vi "Circle Detection Programmattically.vi"(6 "error in":errorcluster, 8 "File Path":path=path "\\\\WS007462\\Share_Station_20/Dinesh/Electrolux/Level 10_11min_4_0001.JPG", 9 "Color Plane (Color Plane Extraction 1)":i32(ring) items=["Red", "Green", "Blue", "Hue", "Saturation", "Luminance", "Value", "Intensity"]) -> (0 "error out":errorcluster, 1 "Number of Circles detected":i32, 2 "Image Out":T1, 3 "Circles (Shape Detection 1)":T2(array[cluster]) {"Position"."Y" format="%.2f"; "Position"."X" format="%.2f"})   [LabVIEW 2020]
uses:
  <vilib>/vision/NI_Vision_Development_Module.lvlib
  <vilib>/vision/Image Controls.llb/IMAQ Image.ctl
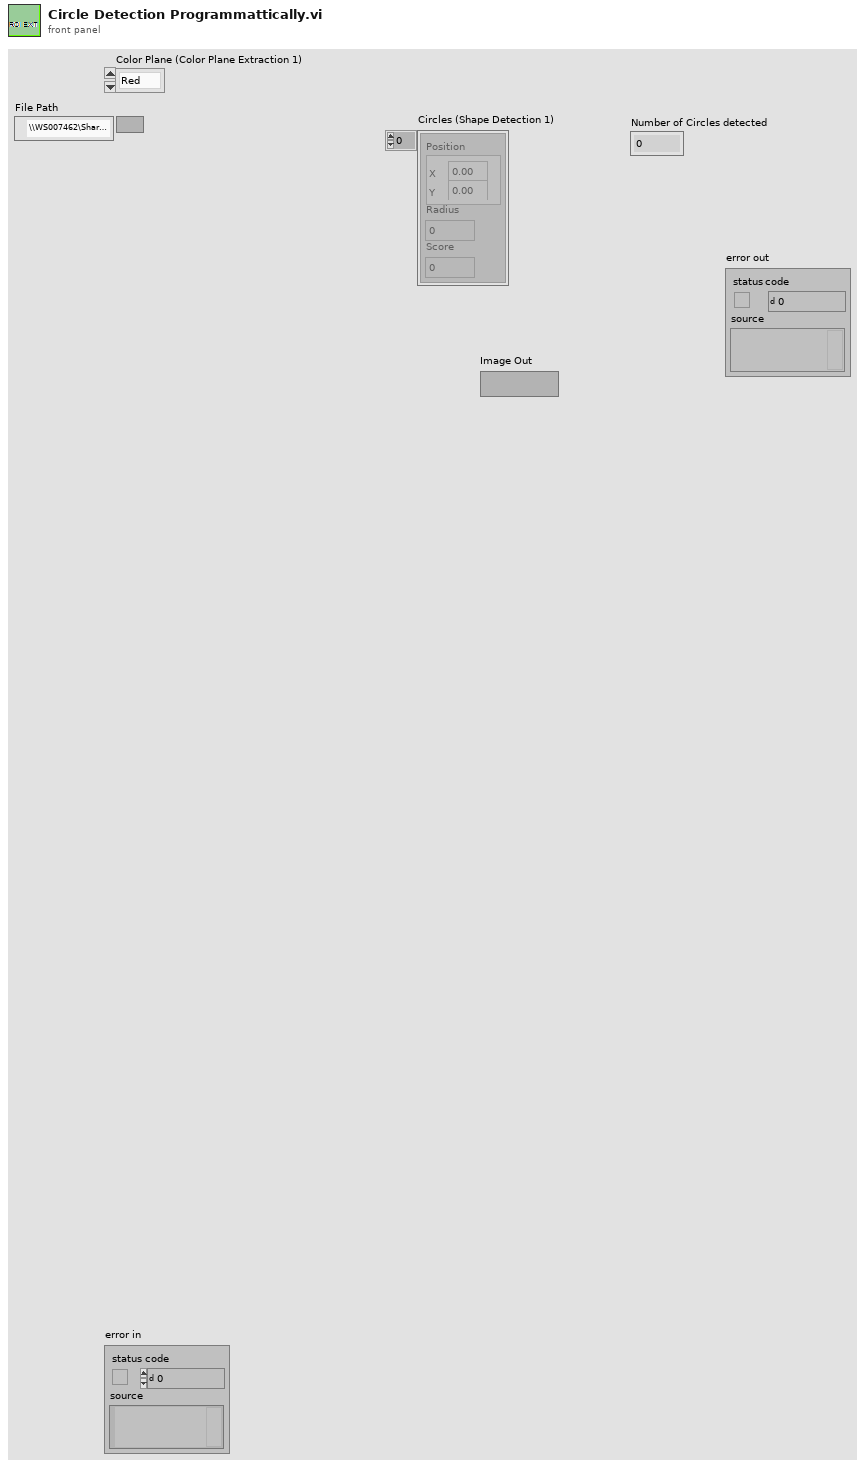
[diagram p1: front panel]
types:
  T1 = typedef "IMAQ Image.ctl" = refnum<image>
  T2 = cluster{"Position":cluster{"X":sgl, "Y":sgl}, "Radius":dbl, "Score":dbl}[]
  T3 = typedef "Image Type" = u32
  T4 = typedef "IMAQ Circle" = cluster{"Center X":i32, "Center Y":i32, "Inner Radius":i32, "Outer Radius":i32, "Start Angle":dbl, "End Angle":dbl}
  T5 = typedef "ROI Descriptor" = cluster{"Global Rectangle":i32[], "Contours":cluster{"ID":enum32{"External", "Internal"}, "Type":u32, "Coordinates":i32[]}[]}
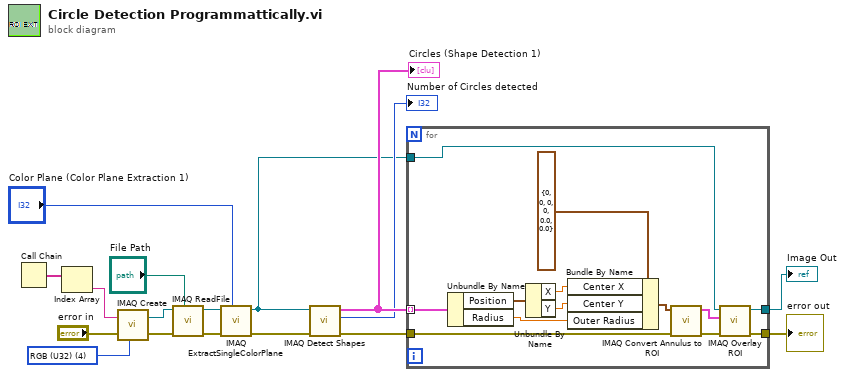
[diagram p0: block diagram]
diagram:
  w11 = T3 4 items=["Grayscale (U8)", "Grayscale (I16)", "Grayscale (SGL)", "Complex (CSG)", "RGB (U32)", "HSL (U32)", "RGB (U64)", "Grayscale (U16)"] ("Image Type")
  n1 = Call Chain() -> (call chain=w13:string[])
  n2 = Index Array(array=w13) -> (element=w12:string)  [unwired: 1 in]
  n3 = call "IMAQ Create"("Image Name"=w12, "Image Type"=w11, "error in (no error)"="error in") -> ("New Image"=w16:T1, "error out"=w15:errorcluster)  [unwired: 1 in, 1 out]
  n4 = call "IMAQ ReadFile"("File Path"="File Path", "error in (no error)"=w15, "Image"=w16) -> ("error out"=w17:errorcluster, "Image Out"=w9:T1)  [unwired: 2 in, 5 out]
  n5 = call "IMAQ ExtractSingleColorPlane"("Color Plane"="Color Plane (Color Plane Extraction 1)", "error in (no error)"=w17, "Image Src"=w9) -> ("error out"=w6:errorcluster, "Image Dst Out"=w3:T1)  [unwired: 1 in, 6 out]
  n6 = call-poly "IMAQ Detect Shapes"("error in (no error)"=w6, "Image"=w3) -> ("error out"=w5:errorcluster, "Number of Matches Returned"=→"Number of Circles detected":i32, "Circles"=w7:T2)  [unwired: 5 in, 2 out]
  "Circles (Shape Detection 1)" <- w7
  n7 = for {
    tunnel: w7 -> [w21] mode=indexing
    tunnel: w5 -> [w24]
    tunnel: w3 -> [w20]
    tunnel: [w19] -> w2
    tunnel: [w18] -> w1
    n8 = Unbundle By Name(w21) -> ("Position"=w28:cluster{"X":sgl, "Y":sgl}, "Radius"=w25:dbl)
    n9 = Unbundle By Name(w28) -> ("X"=w27:sgl, "Y"=w26:sgl)
    n10 = Bundle By Name(cluster=T4 {"Center X"=0, "Center Y"=0, "Inner Radius"=0, "Outer Radius"=0, "Start Angle"=0.0, "End Angle"=0.0} ("Annulus"), "Center X"=w27, "Center Y"=w26, "Outer Radius"=w25) -> (w30:T4)
    n11 = call "IMAQ Convert Annulus to ROI"("error in (no error)"=w24, "Annulus"=w30) -> ("error out"=w22:errorcluster, "ROI Descriptor"=w23:T5)  [unwired: 7 in]
    n12 = call "IMAQ Overlay ROI"("error in (no error)"=w22, "ROI Descriptor"=w23, "Image"=w20) -> ("error out"=w19:errorcluster, "Image Out"=w18:T1)  [unwired: 7 in]
  }
  "error out" <- w2
  "Image Out" <- w1
